vi "Update Speed Ctl.vi"(8 "error in (no error)":errorcluster, 9 "Speed":refnum<vi>, 10 "Step":refnum<vi>, 11 "index":i32) -> (0 "error out":errorcluster, 1 "Speed (dup)":refnum<vi>, 2 "Step (dup)":refnum<vi>)   [LabVIEW 2010, in "SignalWriterMH110203USBStepperMotor.lvclass"]
uses:
  SignalWriterMH110203USBStepperMotor.lvclass
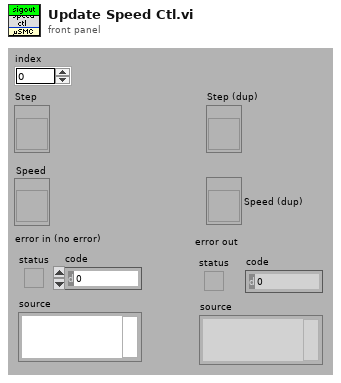
[diagram p1: front panel]
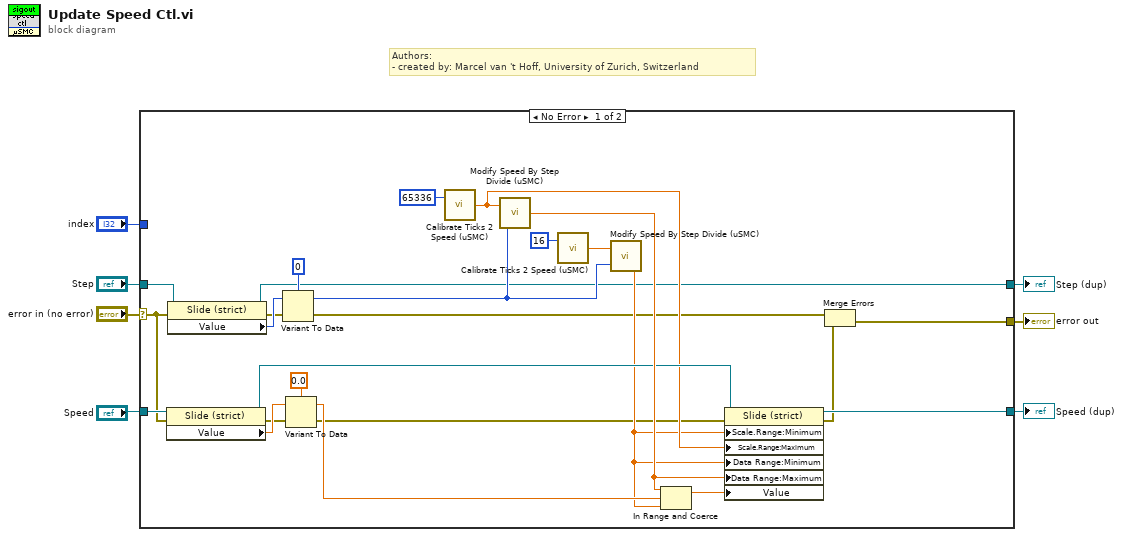
[diagram p0: block diagram]
diagram:
  # "Authors: \n- created by: Marcel van 't Hoff, University of Zurich, Switzerland"
  n1 = case shown="No Error" "error in (no error)" {
    selector: "error in (no error)" -> [w12 w35]
    tunnel: "Speed" -> [w30 w33]
    tunnel: "index" -> [_ _]
    tunnel: "Step" -> [w26 w34]
    tunnel: [w17 w33] -> w1
    tunnel: [w16 w34] -> w2
    tunnel: [w9 w35] -> w5
    frame No Error {
      n2 = property class="Slide (strict)"(reference=w30, error in=w12) -> (reference out=w31:refnum<vi>, error out=w15:errorcluster, "Value"=w21:dbl)
      n3 = property class="Slide (strict)"(reference=w26, error in=w12) -> (reference out=w16:refnum<vi>, error out=w14:errorcluster, "Value"=w24:u8)
      n4 = Variant To Data(error in=w14, Variant=w24, type=u8 0 ("U8 constant")) -> (error out=w11:errorcluster, data=w23:u8)
      n5 = Variant To Data(error in=w15, Variant=w21, type=0.0 ("double constant")) -> (error out=w13:errorcluster, data=w20:dbl)
      n6 = call "Calibrate Ticks 2 Speed (uSMC).vi"("speed ticks"=u16 65336) -> ("speed value (units)"=w25:dbl)  [unwired: 1 in]
      n7 = call "Modify Speed By Step Divide (uSMC).vi"("Step"=w23, "Speed"=w25) -> ("speed"=w32:dbl)
      n8 = call "Calibrate Ticks 2 Speed (uSMC).vi"("speed ticks"=u16 16) -> ("speed value (units)"=w28:dbl)  [unwired: 1 in]
      n9 = call "Modify Speed By Step Divide (uSMC).vi"("Step"=w23, "Speed"=w28) -> ("speed"=w18:dbl)
      n10 = In Range and Coerce(upper limit=w32, x=w20, lower limit=w18) -> (coerced(x)=w8:dbl)  [unwired: 1 out]
      n11 = property on="Property Node" class="Slide (strict)"(reference=w31, error in=w13, "Scale.Range:Minimum"=w18, "Scale.Range:Maximum"=w25, "Data Range:Minimum"=w18, "Data Range:Maximum"=w32, "Value"=w8) -> (reference out=w17:refnum<vi>, error out=w10:errorcluster)
      n12 = Merge Errors(w11, w10) -> (w9:errorcluster)
    }
    frame Error {
    }
  }
  "error out" <- w5
  "Step (dup)" <- w2
  "Speed (dup)" <- w1
